vi "Write Number of Channels.vi"(8 "error in (no error)":errorcluster, 10 "# Channels":u8=2, 11 "Function Generator in":refnum<class "Function Generator.lvclass">) -> (0 "error out":errorcluster, 3 "Function Generator out":refnum<class "Function Generator.lvclass">)   [LabVIEW 2018, in "Function Generator.lvlib" / "Function Generator.lvclass"]
uses:
  Function Generator.lvclass
  Function Generator.lvclass/Function Generator.ctl
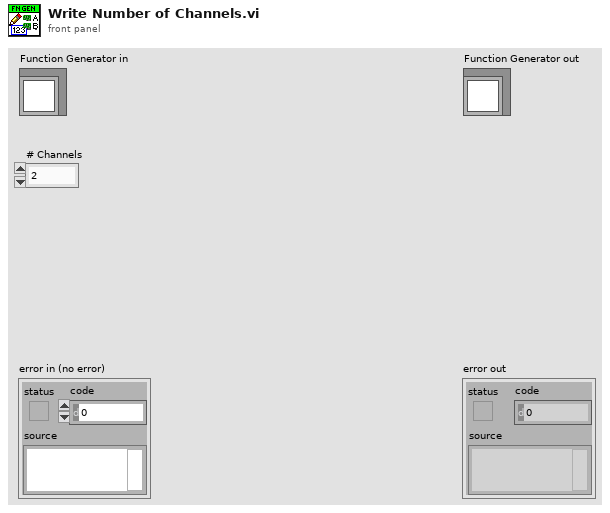
[diagram p1: front panel]
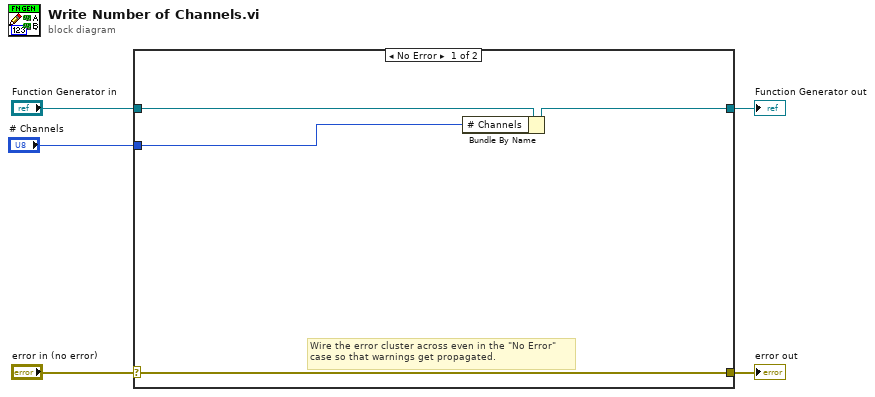
[diagram p0: block diagram]
diagram:
  n1 = case shown="No Error" "error in (no error)" {
    selector: "error in (no error)" -> [w8 w11]
    tunnel: [w8 w11] -> w4
    tunnel: [w7 w10] -> w2
    tunnel: "Function Generator in" -> [w9 w10]
    tunnel: "# Channels" -> [w6 _]
    frame No Error {
      # "Wire the error cluster across even in the \"No Error\"\ncase so that warnings get propagated."
      n2 = Bundle By Name(cluster=w9, "# Channels"=w6) -> (w7:refnum<class "Function Generator.lvclass">)
    }
    frame Error {
    }
  }
  "error out" <- w4
  "Function Generator out" <- w2
